vi "GetNumber.vi"(8 "error in (no error)":errorcluster, 11 "TouchScreen in":refnum<class "TouchScreen.lvclass">) -> (0 "error out":errorcluster, 2 "number":string, 3 "TouchScreen out":refnum<class "TouchScreen.lvclass">)   [LabVIEW 2020, in "TouchScreen.lvlib" / "TouchScreen.lvclass"]
uses:
  TouchScreen.lvclass
  NumPad2/NPad2/NPad2.lvclass
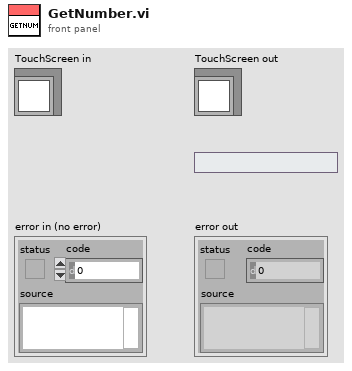
[diagram p1: front panel]
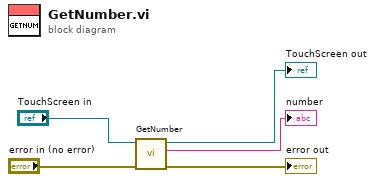
[diagram p0: block diagram]
diagram:
  n1 = call-parent "GetNumber.vi"("error in (no error)"="error in (no error)", "NPad2 in"="TouchScreen in") -> ("error out"=→"error out":errorcluster, "number"=→"number":string, "NPad2 out"=→"TouchScreen out":refnum<class "TouchScreen.lvclass">)  [unwired: 7 in]
